vi "lv9_daqusb6251.vi"() -> ()   [LabVIEW 2009]
panel:
  out "Final time [s]":dbl
  out "m":dbl
  out "s":dbl
  out "h":dbl
  out "Iteration":i32
  out "Waveform Chart 8":dynamicdata(graph)
  out "Waveform Chart 7":dynamicdata(graph)
  out "Waveform Chart 6":dynamicdata(graph)
  out "Waveform Chart 5":dynamicdata(graph)
  out "Waveform Chart 4":dynamicdata(graph)
  out "Waveform Chart 3":dynamicdata(graph)
  out "Waveform Chart 2":dynamicdata(graph)
  in  "Device name":tag
  in  "Number of samples \nto read":i32
  in  "Acquisition rate [Hz]":dbl
  out "Waveform Chart":dynamicdata(graph)
  in  "Stop":bool
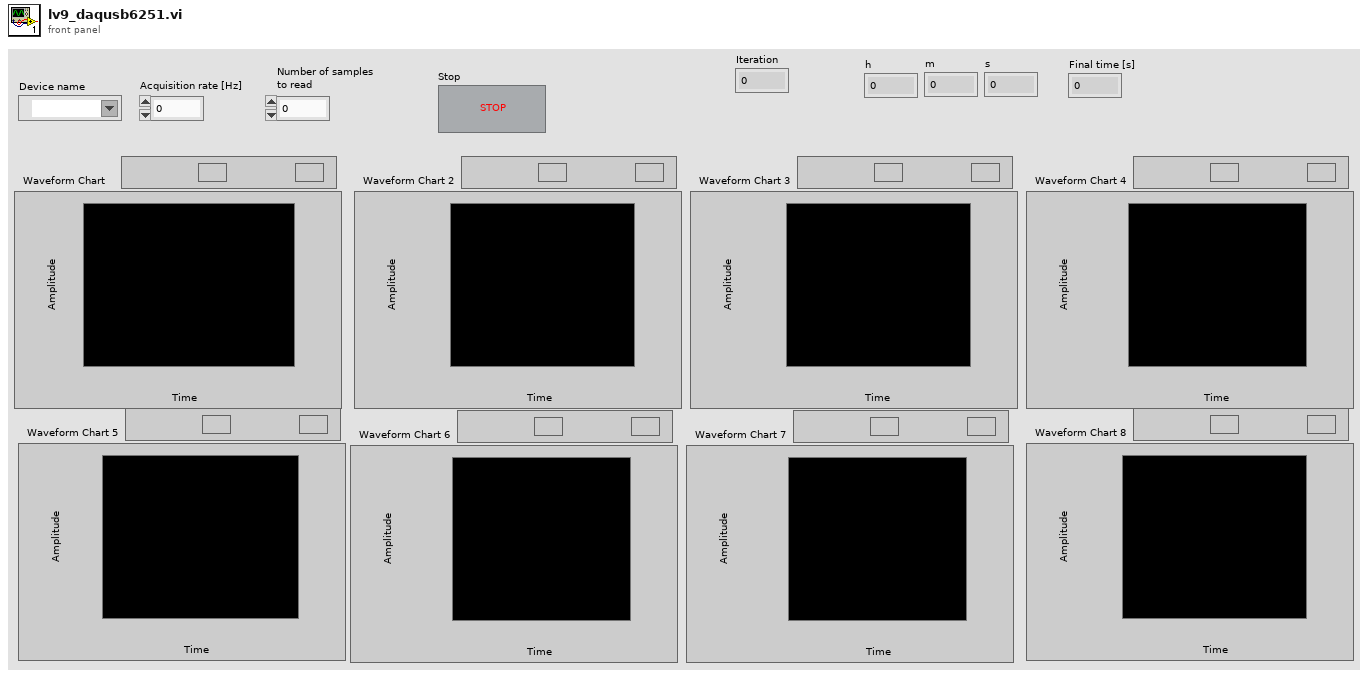
[diagram p1: front panel]
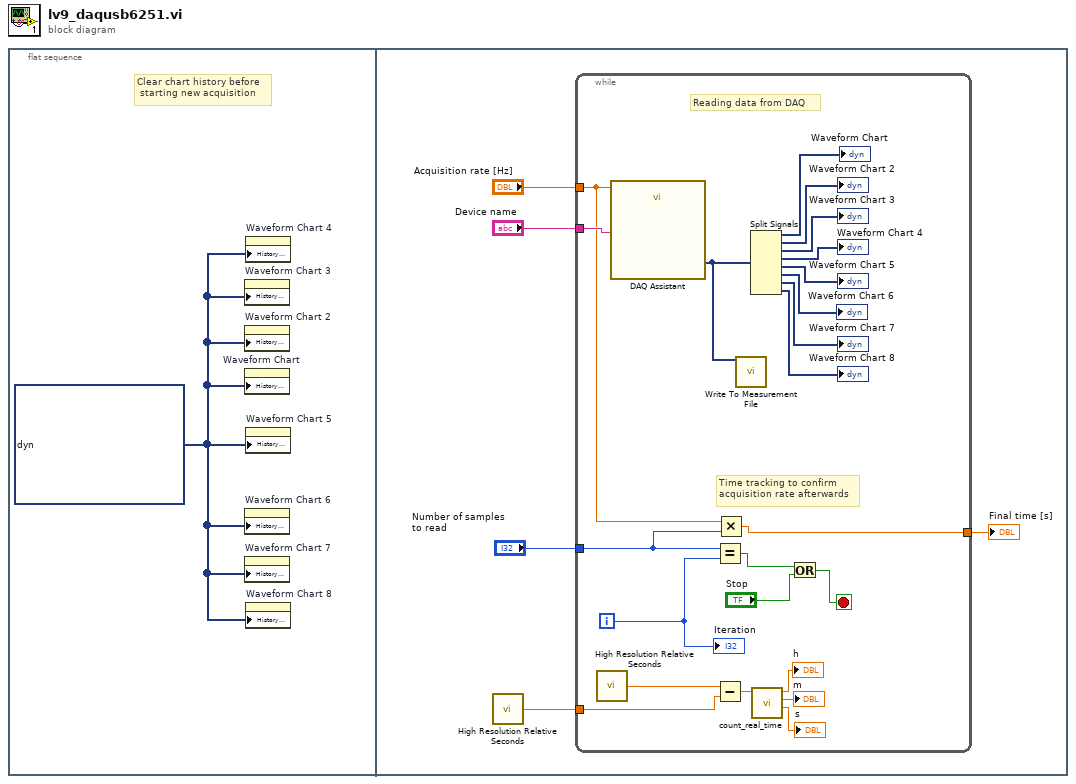
[diagram p0: block diagram]
diagram:
  n1 = flat-sequence {
    frame #0 {
      w1 = dynamicdata[] ? ("History Data")
      # "Clear chart history before\n starting new acquisition"
      n2 = property on="Waveform Chart 3" class="WFChart (strict)"("History Data"=w1) -> ()  [unwired: 2 in, 2 out]
      n3 = property on="Waveform Chart 2" class="WFChart (strict)"("History Data"=w1) -> ()  [unwired: 2 in, 2 out]
      n4 = property on="Waveform Chart" class="WFChart (strict)"("History Data"=w1) -> ()  [unwired: 2 in, 2 out]
      n5 = property on="Waveform Chart 6" class="WFChart (strict)"("History Data"=w1) -> ()  [unwired: 2 in, 2 out]
      n6 = property on="Waveform Chart 7" class="WFChart (strict)"("History Data"=w1) -> ()  [unwired: 2 in, 2 out]
      n7 = property on="Waveform Chart 4" class="WFChart (strict)"("History Data"=w1) -> ()  [unwired: 2 in, 2 out]
      n8 = property on="Waveform Chart 5" class="WFChart (strict)"("History Data"=w1) -> ()  [unwired: 2 in, 2 out]
      n9 = property on="Waveform Chart 8" class="WFChart (strict)"("History Data"=w1) -> ()  [unwired: 2 in, 2 out]
    }
    frame #1 {
      n10 = call <vilib>:"High Resolution Relative Seconds.vi"() -> ("relative seconds"=w5:dbl)
      n11 = while {
        tunnel: "Device name" -> [w28]
        tunnel: "Number of samples \nto read" -> [w15]
        tunnel: [w14] -> w4
        tunnel: w5 -> [w8]
        tunnel: "Acquisition rate [Hz]" -> [w7]
        i -> [w17]
        stop <- w18 stop-if-true
        # "Reading data from DAQ"
        # "Time tracking to confirm\nacquisition rate afterwards"
        n12 = call <vilib>:"High Resolution Relative Seconds.vi"() -> ("relative seconds"=w13:dbl)
        n13 = call "DAQ Assistant"("rate"=w7, "device name"=w28) -> ("data"=w27:dynamicdata)  [unwired: 14 in, 3 out]
        n14 = Equal?(x=w15, y=w17) -> (x = y?=w16:bool)
        n15 = Subtract(x=w13, y=w8) -> (x-y=w12:dbl)
        n16 = Multiply(x=w7, y=w15) -> (x*y=w14:dbl)
        n17 = call "Write To Measurement File"("Signals"=w27) -> ()  [unwired: 16 in, 3 out]
        n18 = Split Signals(w27) -> (→"Waveform Chart":dynamicdata, →"Waveform Chart 2":dynamicdata, →"Waveform Chart 3":dynamicdata, →"Waveform Chart 4":dynamicdata, →"Waveform Chart 5":dynamicdata, →"Waveform Chart 6":dynamicdata, →"Waveform Chart 7":dynamicdata, →"Waveform Chart 8":dynamicdata)  [unwired: 8 in]
        n19 = call "count_real_time.vi"("Total time in seconds"=w12) -> ("Sec"=→"s":dbl, "Min"=→"m":dbl, "H"=→"h":dbl)  [unwired: 8 in]
        n20 = Or(x=w16, y="Stop") -> (x .or. y?=w18:bool)
        "Iteration" <- w17
      }
      "Final time [s]" <- w4
    }
  }
